vi "sequence util_audit.vi"(8 "error in":errorcluster, 9 "Item Names IN":string[](array[string])=["----------    AH Bridge: Save GPIB address   ", "Write to VISA, GPIB::27::INSTR, FILE STORE GPIB USERPON", "----------    LakeShore 340 controller: change heater power (0-5, 0: off)  ", "Write to VISA, GPIB::12::INSTR, RANGE 0", "----------    Scheduled T-control for the He3 system   ", "Wait for 12 hour", "Set Temperature LS336 ( GPIB0::12::INSTR ) 45 K at 0 K/min, Output 1", "Wait for 60 s", "Wait for Temperature Less than 1.8 K Sensor C of LS336 ( GPIB0::14::INSTR ) Timeout 30 min", "Wait for 60 min", "Set Temperature LS336 ( GPIB0::12::INSTR ) 0.1 K at 0 K/min, Output 1", "----------    Motor control (use Instrumet:Set:MotorControl command structure)  ", "Set MotorControl ( BLM ) 12345 0.2", "Wait for VI value localhost, BLM_ManualControl.vi, BLM Position, Within, 12345, 10 min", "Wait for 10 s", "END SEQUENCE"]) -> (0 "error out":errorcluster, 1 "Item Names out":string[](array[string]))   [LabVIEW 2021]
panel:
  out "progress (%)":i32
  out "# of warnings":i32
  out "# of errors":i32
  out "Array":dbl[][][](array[numeric])
  in  "highlight line contains following text":cluster{"String":string, "Color Box":u32}[](array[cluster])
  out "XY Graph":cluster{dbl[], dbl[]}[](graph)
  in  "commands identifier":string[][](array[string])=[["Set Field", "T", " "], ["Set Temperature", "K", ")"], ["Set MotorControl", ":", " "]]
  in  "file (use dialog)":path
  in  "expand macro":bool
  in  "sequence in":i32(listbox)
  in  "Cancel":bool
  in  "Done":bool
  # "(can be edited for root commands (commands not in the subsequence))"
  # "non-parameter constant"
  # "string before parameter"
  # "string after parameter"
  # "XY Graph plots parameter of a specific commands as a function of line number.\n\nThe command is identified by 'head string' and strings right after (usually unit)\n and before the command structure.\n\nFor non-parameter commands, such as 'Stop', 'Start', use the non-parameter constant \nas a fake parameter to identify them easily. Otherwise, those commands appear as 0."
  # "If expand macro is ON, sequences are labelled #.n (n= 0 for main command, n>0 for expanded command)."
  # "under construction"
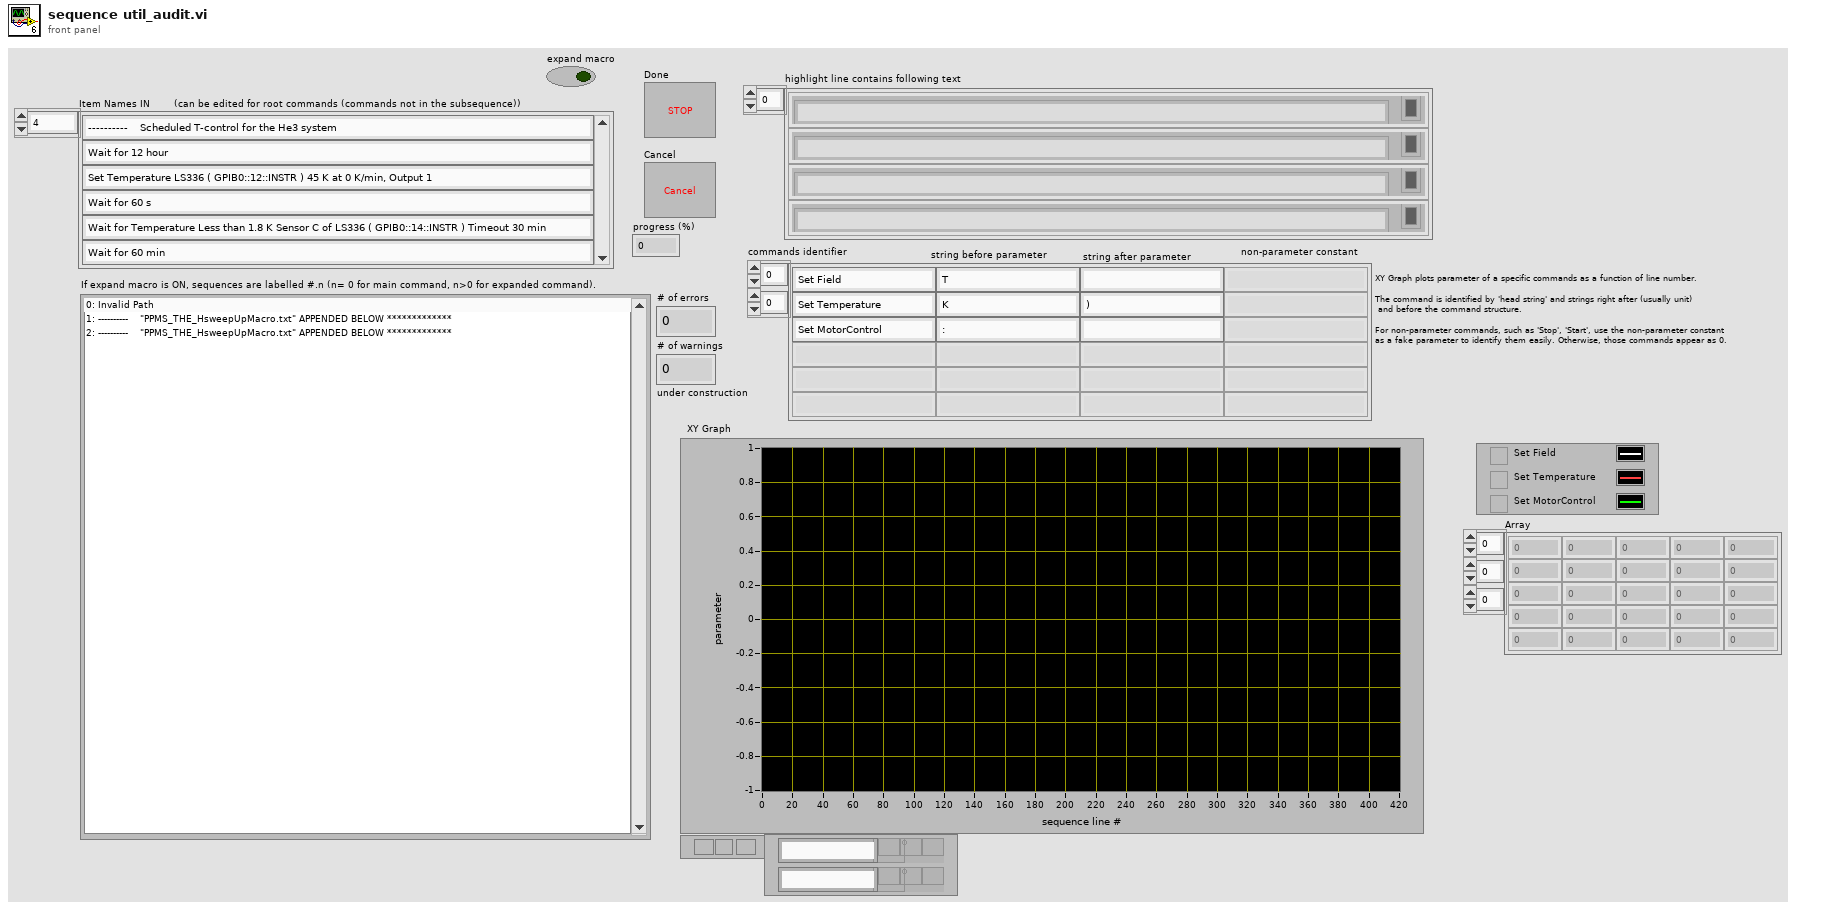
[diagram p1: front panel]
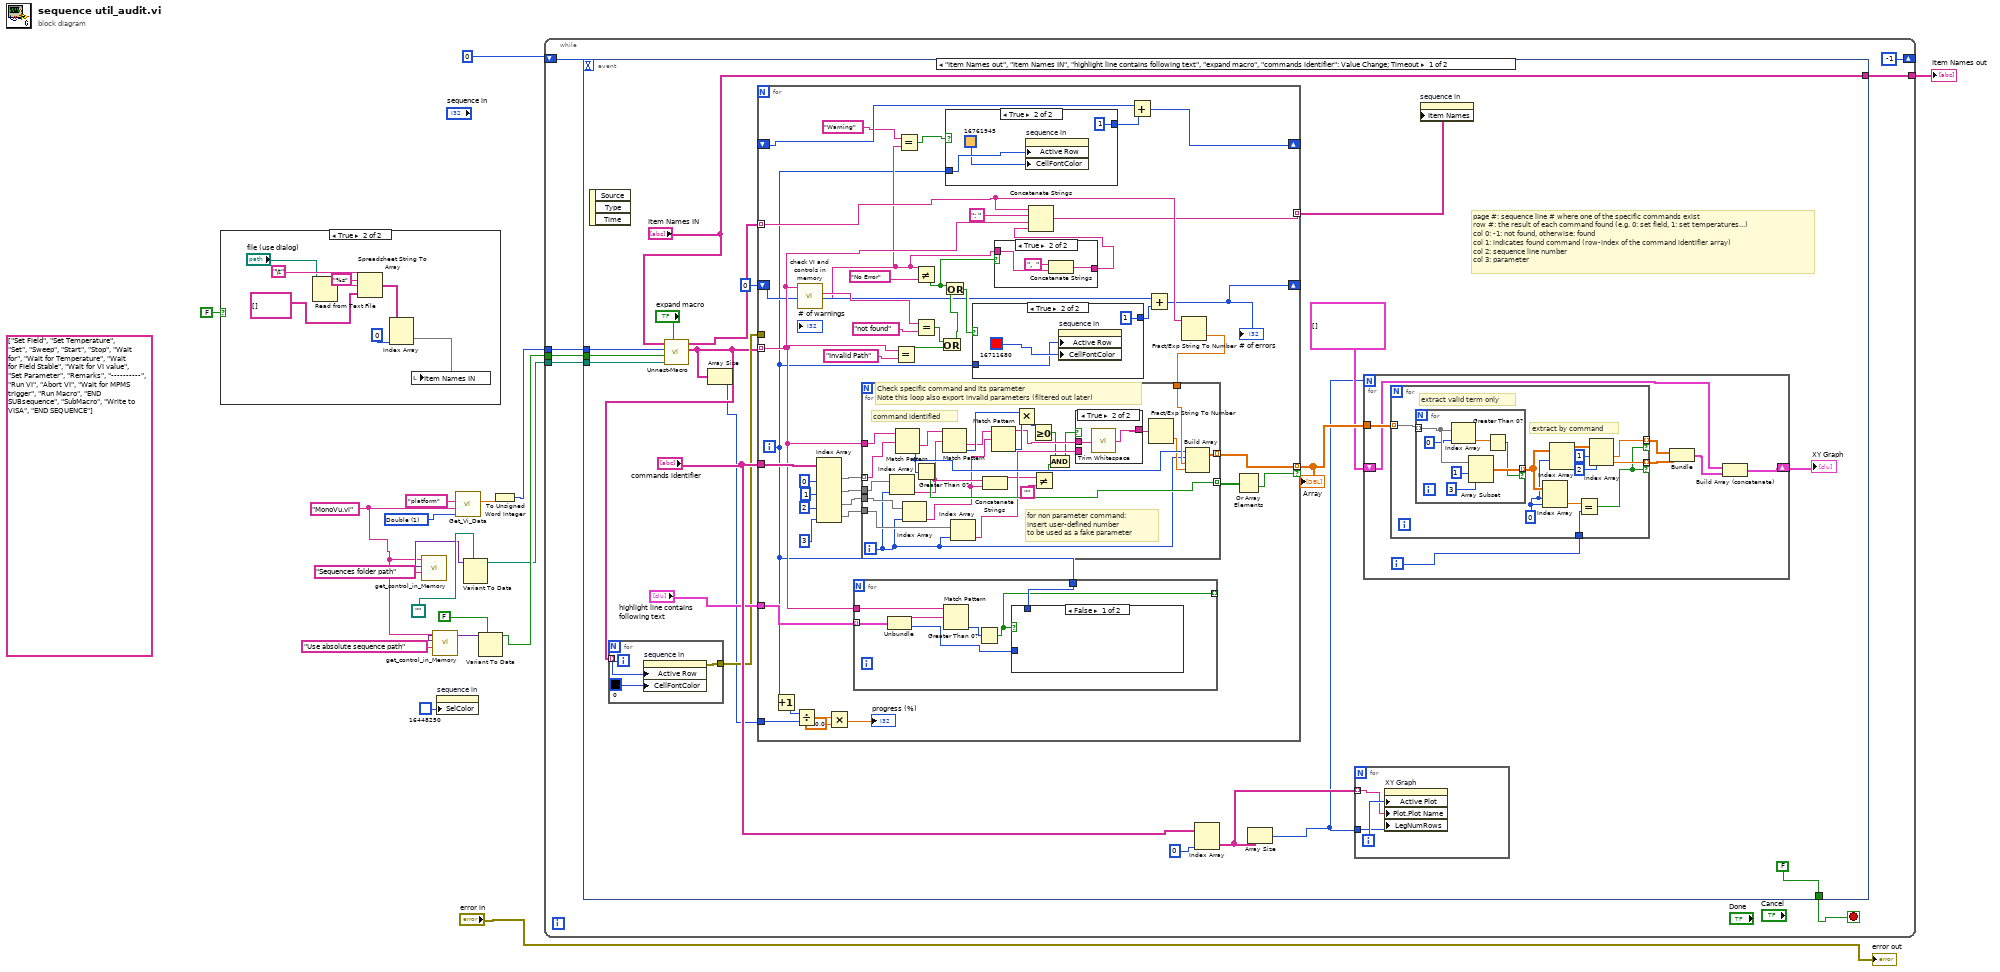
[diagram p0: block diagram]
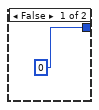
[diagram p2: hidden frame]
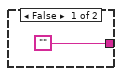
[diagram p3: hidden frame]
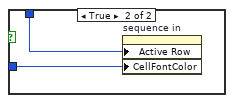
[diagram p4: hidden frame]
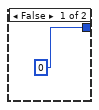
[diagram p6: hidden frame]
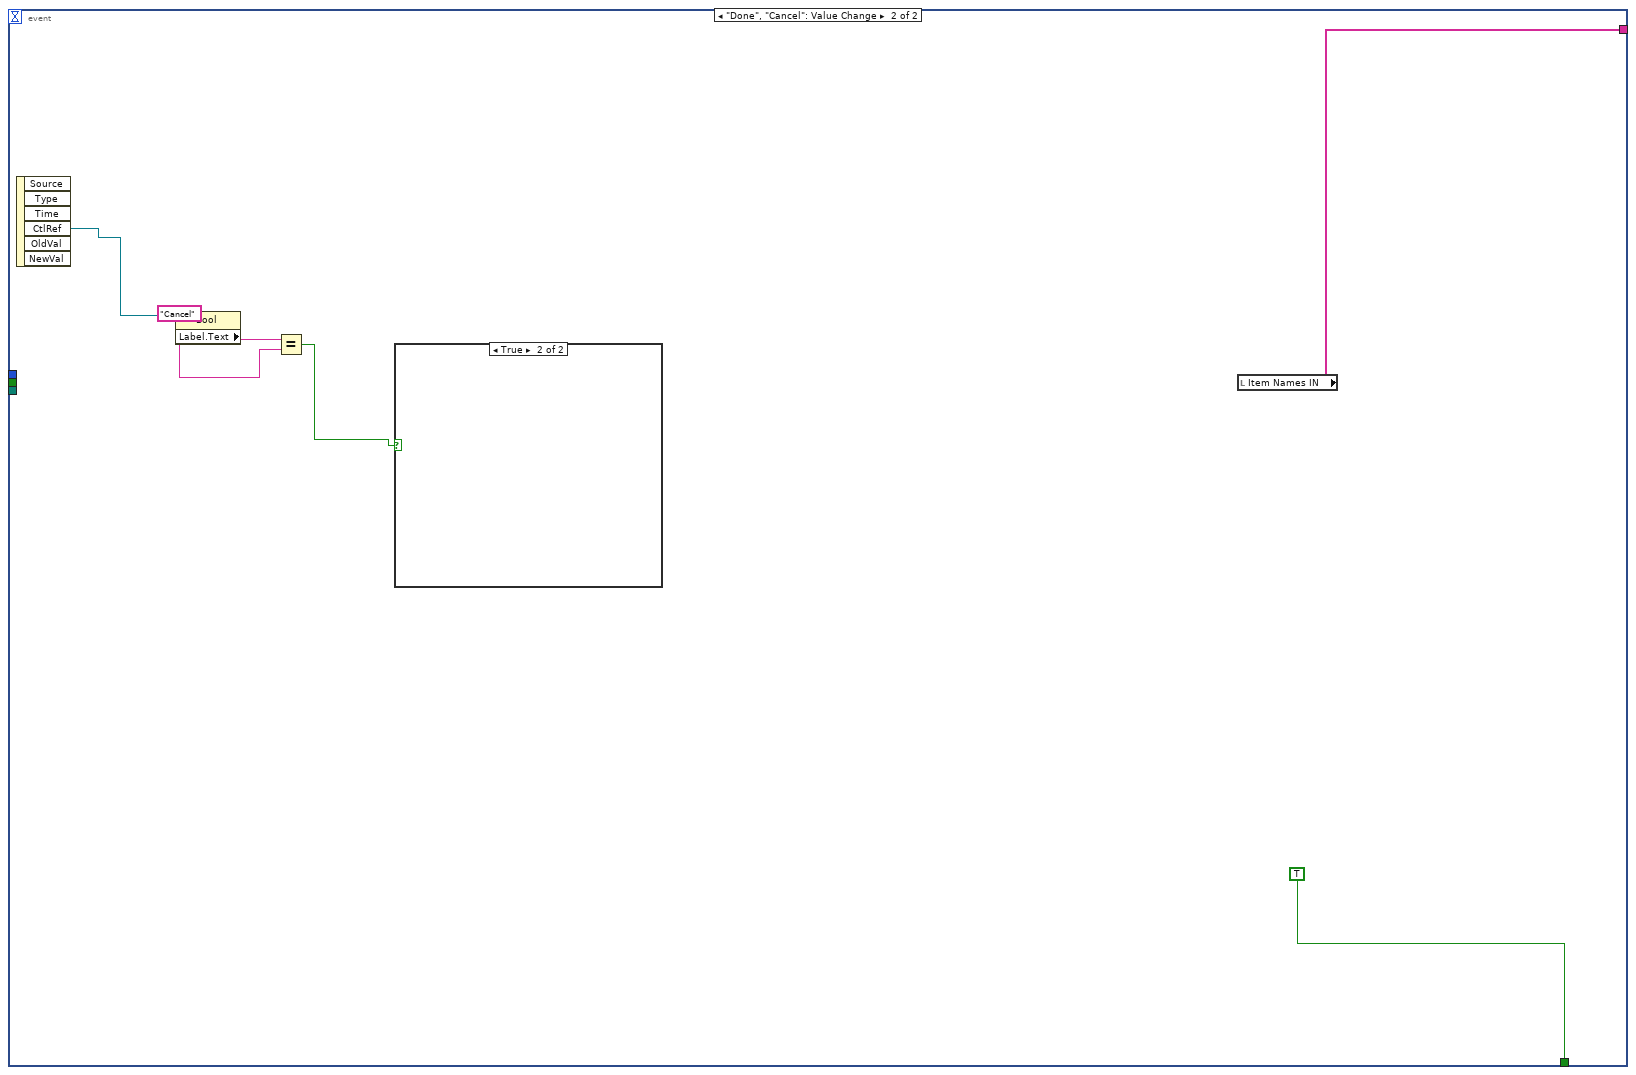
[diagram p7: hidden frame]
diagram:
  w13 = u16 1 items=["String", "Double", "Boolean", "Variant"] ("Data Type")
  w4 = "MonoVu.vi" ("VI Name")
  (unwired) string[] ["Set Field", "Set Temperature", "Set", "Sweep", "Start", "Stop", "Wait for", "Wait for Temperature", "Wait for Field Stable", "Wait for VI value", "Set Parameter", "Remarks", "----------", "Run VI", "Abort VI", "Wait for MPMS trigger", "Run Macro", "END SUBsequence", "SubMacro", "Write to VISA", "END SEQUENCE"] ("command list-all")
  n1 = case shown="True" FALSE {
    frame False {
    }
    frame True {
      n2 = Read from Text File(file (use dialog)="file (use dialog)") -> (text=w26:string)  [unwired: 3 in, 3 out]
      n3 = Spreadsheet String To Array(delimiter (Tab)="\t", format string="%s", spreadsheet string=w26, array type (2D Dbl)=string[][] []) -> (array=w23:string[][])
      n4 = Index Array(array=w23, index (col)=0 ("index (row)")) -> (element=w20:string[])  [unwired: 1 in]
      n5 = local write "Item Names IN"(w20) -> ()
    }
  }
  n6 = call "get_control_in_Memory.vi"("Control Name"="Sequences folder path", "VI Name"=w4) -> ("Value"=w8:variant)  [unwired: 2 in, 1 out]
  n7 = call "get_control_in_Memory.vi"("Control Name"="Use absolute sequence path", "VI Name"=w4) -> ("Value"=w5:variant)  [unwired: 2 in, 1 out]
  n8 = property on="sequence in" class="LstBox (strict)"("SelColor"=u32 16448250 ("Selection Color")) -> ()  [unwired: 2 in, 2 out]
  n9 = call "Get_Vi_Data.vi"("Data Type"=w13, "VI name"=w4, "Control Name"="platform") -> ("Data (Double)"=w11:dbl)  [unwired: 4 in, 4 out]
  n10 = Variant To Data(type=path "" ("Path"), Variant=w8) -> (data=w1:path)  [unwired: 1 in, 1 out]
  n11 = Variant To Data(type=FALSE ("Use LS336Panel.vi"), Variant=w5) -> (data=w2:bool)  [unwired: 1 in, 1 out]
  n12 = To Unsigned Word Integer(number=w11) -> (unsigned 16bit integer=w3:u16)
  n13 = while {
    shift-right: [-1 ("sequence in")] -> _
    shift-left: 0 ("sequence in") -> [w32]
    tunnel: [w30] -> w14
    tunnel: w3 -> [w29]
    tunnel: w2 -> [w28]
    tunnel: w1 -> [w27]
    stop <- w33 stop-if-true
    n14 = event shown="[0] \"Item Names out\", \"Item Names IN\", \"highlight line contains following text\", \"expand macro\", \"commands identifier\": Value Change;  Timeout" {
      selector: _ -> [_ _]
      dyn-events: _ -> [_ _]
      timeout: w32 -> [_ _]
      tunnel: [FALSE TRUE] -> w33
      tunnel: ["Item Names IN" w178] -> w30
      tunnel: w29 -> [w36 _]
      tunnel: w28 -> [w35 _]
      tunnel: w27 -> [w34 _]
      event "Item Names out", "Item Names IN", "highlight line contains following text", "expand macro", "commands identifier": Value Change; Timeout {
        # "page #: sequence line # where one of the specific commands exist\nrow #: the result of each command found (e.g. 0: set field, 1: set temperatures...)\ncol 0: -1: not found, otherwise: found\ncol 1: indicates found command (row-index of the command identifier array)\ncol 2: sequence line number\ncol 3: parameter"
        n15 = event-data() -> ()  [unwired: 1 in, 3 out]
        n16 = call "Unnest-Macro.vi"("expand"="expand macro", "Sequences folder path"=w34, "Use absolute sequence path"=w35, "platform"=w36, "Item Names IN"="Item Names IN") -> ("unnested items"=w38:string[], "item index"=w43:string[])  [unwired: 5 in]
        n17 = for {
          tunnel: w38 -> [_] mode=indexing
          tunnel: [w54] -> w42
          i -> [w56]
          n18 = property on="sequence in" class="LstBox (strict)"("Active Row"=w56, "CellFontColor"=u32 0 ("Active Row:Cell Font:Color")) -> (error out=w54:errorcluster)  [unwired: 2 in, 1 out]
        }
        n19 = Array Size(array=w38) -> (size(s)=w37:i32)
        n20 = for {
          tunnel: w38 -> [w106] mode=indexing
          tunnel: [w124] -> w52 mode=indexing
          tunnel: [w116] -> w51 mode=indexing if=w110
          tunnel: w43 -> [w126] mode=indexing
          tunnel: "commands identifier" -> [w123]
          tunnel: "highlight line contains following text" -> [w113]
          tunnel: w42 -> [_]
          shift-right: [w97] -> _
          shift-left: 0 -> [w98]
          shift-right: [w95] -> _
          shift-left: _ -> [w94]
          tunnel: w37 -> [w89]
          i -> [w90]
          n21 = Increment(x=w90) -> (x+1=w85:i32)
          n22 = Divide(x=w85, y=w89) -> (x/y=w88:dbl)
          n23 = call "check VI and controls in memory.vi"("Input command"=w106) -> ("error message"=w93:string, "Identifield command"=w105:string)  [unwired: 7 in, 2 out]
          n24 = Index Array(array=w123, index (col) #1=0 ("disabled index (col)"), index (col) #2=1 ("index (col)"), index (col) #3=2 ("index (col)"), index (col) #4=3 ("index (col)")) -> (element #1=w120:string[], element #2=w119:string[], element #3=w114:string[], element #4=w111:string[])  [unwired: 4 in]
          n25 = Multiply(x=w88, y=100.0) -> (x*y=→"progress (%)":dbl)
          n26 = for {
            tunnel: w113 -> [w140] mode=indexing
            tunnel: w106 -> [w142]
            tunnel: w90 -> [w137]
            tunnel: [w136] -> _ mode=indexing
            n27 = Unbundle(w140) -> ("String"=w139:string, "Color Box"=w138:u32)
            n28 = Match Pattern(string=w142, regular expression=w139) -> (offset past match=w141:i32)  [unwired: 1 in, 3 out]
            n29 = Greater Than 0?(x=w141) -> (x > 0?=w136:bool)
            n30 = case shown="False" w136 {
              tunnel: w138 -> [_ w143]
              tunnel: w137 -> [_ w144]
              frame False {
              }
              frame True {
                n31 = property on="sequence in" class="LstBox (strict)"("Active Row"=w144, "CellFontColor"=w143) -> ()  [unwired: 2 in, 2 out]
              }
            }
          }
          n32 = Equal?(x=w106, y="Invalid Path") -> (x = y?=w107:bool)
          n33 = Equal?(x="Warning" ("y"), y=w93) -> (x = y?=w91:bool)
          n34 = Not Equal?(x=w93, y="No Error") -> (x != y?=w101:bool)
          n35 = Equal?(x=w105, y="not found") -> (x = y?=w108:bool)
          n36 = Or(x=w108, y=w107) -> (x .or. y?=w103:bool)
          n37 = Or(x=w101, y=w103) -> (x .or. y?=w102:bool)
          n38 = case shown="True" w91 {
            tunnel: w90 -> [_ w130]
            tunnel: [0 1] -> w96
            frame False {
            }
            frame True {
              n39 = property on="sequence in" class="LstBox (strict)"("Active Row"=w130, "CellFontColor"=u32 16761945 ("Active Row:Cell Font:Color")) -> ()  [unwired: 2 in, 2 out]
            }
          }
          n40 = case shown="True" w102 {
            tunnel: w90 -> [_ w176]
            tunnel: [0 1] -> w99
            frame False {
            }
            frame True {
              n41 = property on="sequence in" class="LstBox (strict)"("Active Row"=w176, "CellFontColor"=u32 16711680 ("Active Row:Cell Font:Color")) -> ()  [unwired: 2 in, 2 out]
            }
          }
          n42 = case shown="True" w101 {
            tunnel: ["" w135] -> w100
            tunnel: w93 -> [_ w134]
            frame False {
            }
            frame True {
              n43 = Concatenate Strings(",  " ("string"), w134) -> (w135:string)
            }
          }
          n44 = Concatenate Strings(w126, ": ", w106, w100) -> (w124:string)
          n45 = Add(x=w94, y=w96) -> (x+y=w95:i32)
          n46 = Add(x=w98, y=w99) -> (x+y=w97:i32)
          "# of errors" <- w97
          n47 = Fract/Exp String To Number(string=w126) -> (number=w117:dbl)  [unwired: 3 in, 1 out]
          n48 = for {
            tunnel: [w165] -> w118 mode=indexing
            tunnel: w106 -> [w166]
            tunnel: w120 -> [w169] mode=indexing
            tunnel: w119 -> [w158]
            tunnel: w117 -> [w167]
            tunnel: [w168] -> w116 mode=indexing
            tunnel: w114 -> [w156]
            tunnel: w111 -> [w157]
            i -> [w155]
            # "for non parameter command:\ninsert user-defined number\nto be used as a fake parameter"
            # "command identified"
            # "Check specific command and its parameter\nNote this loop also export invalid parameters (filtered out later)"
            n49 = Index Array(array=w158, index=w155) -> (element=w150:string)
            n50 = Match Pattern(string=w166, regular expression=w169) -> (after substring=w170:string, offset past match=w164:i32)  [unwired: 1 in, 2 out]
            n51 = Index Array(array=w156, index=w155) -> (element=w149:string)
            n52 = Greater Than 0?(x=w164) -> (x > 0?=w165:bool)
            n53 = Match Pattern(string=w170, regular expression=w150) -> (after substring=w153:string, offset past match=w161:i32)  [unwired: 1 in, 2 out]
            n54 = Index Array(array=w157, index=w155) -> (element=w154:string)
            n55 = Concatenate Strings(w150, w149) -> (w148:string)
            n56 = Match Pattern(string=w153, regular expression=w149) -> (before substring=w152:string, offset past match=w160:i32)  [unwired: 1 in, 2 out]
            n57 = Multiply(x=w161, y=w160) -> (x*y=w159:i32)
            n58 = Greater Or Equal To 0?(x=w159) -> (x >= 0?=w146:bool)
            n59 = Not Equal?(x=w148, y="") -> (x != y?=w147:bool)
            n60 = And(x=w146, y=w147) -> (x .and. y?=w145:bool)
            n61 = case shown="True" w145 {
              tunnel: w152 -> [_ w173]
              tunnel: [w171 w172] -> w163
              tunnel: w154 -> [w171 _]
              frame False {
              }
              frame True {
                n62 = call <vilib>:"Trim Whitespace.vi"("string"=w173) -> ("trimmed string"=w172:string)  [unwired: 1 in]
              }
            }
            n63 = Fract/Exp String To Number(string=w163) -> (number=w162:dbl)  [unwired: 3 in, 1 out]
            n64 = Build Array(w164, w155, w167, w162) -> (w168:dbl[])
          }
          n65 = Or Array Elements(Boolean array=w118) -> (logical OR=w110:bool)
        }
        "Array" <- w51
        n66 = Index Array(array="commands identifier", index (col)=0 ("disabled index (col)")) -> (element=w47:string[])  [unwired: 1 in]
        n67 = Array Size(array=w47) -> (size(s)=w45:i32)
        n68 = for {
          tunnel: w47 -> [w58] mode=indexing
          tunnel: w45 -> [w57]
          i -> [w59]
          n69 = property on="XY Graph" class="XYGraph (strict)"("Active Plot"=w59, "Plot.Plot Name"=w58, "LegNumRows"=w57) -> ()  [unwired: 2 in, 2 out]
        }
        n70 = for {
          N: w45 -> [_]
          tunnel: w51 -> [w66]
          shift-right: [w61] -> w49
          shift-left: cluster{dbl[], dbl[]}[] [] -> [w60]
          i -> [w65]
          n71 = for {
            tunnel: w66 -> [w77] mode=indexing
            tunnel: w65 -> [w75]
            tunnel: [w69] -> w64 mode=indexing if=w67
            tunnel: [w68] -> w63 mode=indexing if=w67
            w73 = 0 ("disabled index (col)")
            # "extract by command"
            # "extract valid term only"
            n72 = for {
              tunnel: w77 -> [w83] mode=indexing
              tunnel: [w80] -> w74 mode=indexing if=w79
              n73 = Index Array(array=w83, index=0) -> (element=w84:dbl)
              n74 = Array Subset(array=w83, index=1, length=3) -> (w80:dbl[])
              n75 = Greater Than 0?(x=w84) -> (x > 0?=w79:bool)
            }
            n76 = Index Array(array=w74, index (row)=w73, index (col)=w73) -> (element=w76:dbl)
            n77 = Index Array(array=w74, index (row)=w73) -> (element=w72:dbl[])  [unwired: 1 in]
            n78 = Equal?(x=w76, y=w75) -> (x = y?=w67:bool)
            n79 = Index Array(array=w72, index #1=1 ("index"), index #2=2 ("index")) -> (element #1=w69:dbl, element #2=w68:dbl)
          }
          n80 = Bundle(w64, w63) -> (w62:cluster{dbl[], dbl[]})  [unwired: 1 in]
          n81 = Build Array (concatenate)(w60, w62) -> (w61:cluster{dbl[], dbl[]}[])
        }
        "XY Graph" <- w49
        n82 = property on="sequence in" class="LstBox (strict)"("Item Names"=w52) -> ()  [unwired: 2 in, 2 out]
      }
      event "Done", "Cancel": Value Change {
        n83 = event-data() -> ("CtlRef"=w182:refnum<vi>)  [unwired: 1 in, 5 out]
        n84 = property class="Bool"(reference=w182) -> ("Label.Text"=w181:string)  [unwired: 1 in, 2 out]
        n85 = Equal?(x=w181, y="Cancel") -> (x = y?=w179:bool)
        n86 = case shown="True" w179 {
          frame False {
          }
          frame True {
          }
        }
        n87 = local read "Item Names IN"() -> (w178:string[])
      }
    }
  }
  "Item Names out" <- w14
  "error out" <- "error in"
